vi "Write u8.vi"(8 "Error In":errorcluster) -> (0 "Error Out":errorcluster)   [LabVIEW 2017, in "Tests.lvlib" / "Writer.lvlib"]
uses:
  Writer.lvlib
  <vilib>/addons/_JKI Toolkits/Caraya/classes/Test/Test.lvclass
  <vilib>/addons/_JKI Toolkits/Caraya/classes/Assert/Assert.lvclass
  src/LabPack/Public/Writer/Writer.lvclass
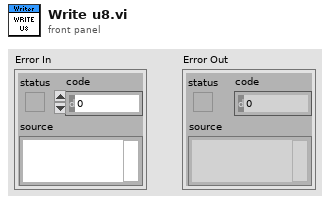
[diagram p1: front panel]
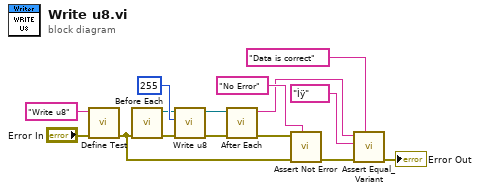
[diagram p0: block diagram]
diagram:
  n1 = call <vilib>:"Define Test.vi"("error in (no error)"="Error In", "Label (VI Title)"="Write u8") -> ("error out"=w11:errorcluster)  [unwired: 9 in]
  n2 = call "Before Each.vi"("Error In"=w11) -> ("Error Out"=w5:errorcluster, "Writer Out"=w4:refnum<class "Writer.lvclass">)  [unwired: 9 in]
  n3 = call "Write u8.vi"("Error In"=w5, "Value"=u8 255, "Writer In"=w4) -> ("Error Out"=w2:errorcluster, "Writer Out"=w3:refnum<class "Writer.lvclass">)  [unwired: 7 in]
  n4 = call "After Each.vi"("Error In"=w2, "Writer In"=w3) -> ("Error Out"=w10:errorcluster, "Data"=w1:string)  [unwired: 8 in]
  n5 = call <vilib>:"Assert Not Error.vi"("Label"="No Error", "error in (no error)"=w11, "Not Error?"=w10) -> ("error out"=w13:errorcluster)  [unwired: 8 in]
  n6 = call <vilib>:"Assert Equal_Variant.vi"("Label"="Data is correct", "error in (no error)"=w13, "Y"="Ìÿ" ("Data"), "X"=w1) -> ("error out"=→"Error Out":errorcluster)  [unwired: 7 in]
